vi "pointer basics.vi"() -> ()   [LabVIEW 2016]
uses:
  API/JSON Document Class/json to string/json To Minimized String - string path.vi
  API/JSON Document Class/JSON Document.lvclass
panel:
  out "error out":errorcluster
  in  "error in (no error)":errorcluster
  out "/pi":string
  out "/foo/1":string
  out "/foo/0":string
  out "/foo":string
  out "null":string
  # "Source JSON"
  # "{\n    \"foo\" : [\"bar\", \"baz\"],\n    \"pi\" : 3.1416\n}"
  # "This VI shows the basics of the pointer format.\nThe source JSON is flattened to a string at each pointer.\nrapidJSON supports String representations. Additionally, it fully supports RFC6901 also defines the URI fragment representation of JSON pointer. URI fragment is specified in RFC3986 \"Uniform Resource Identifier (URI): Generic Syntax\".\n\nThe main differences are that a the URI fragment always has a # (pound sign) in the beginning, and some characters are encoded by percent-encoding in UTF-8 sequence. For example, the following table shows different C/C++ string literals of different representations.\n\nIt additionally can accept an array of tokens"
  # "Providing the path to a key in an object return the value of that object"
  # "Providing null or an empty string returns the entire structure"
  # "Providing the path to an array element returns the element at that index"
  # "Structured types can be nested, e.g. an array inside an object."
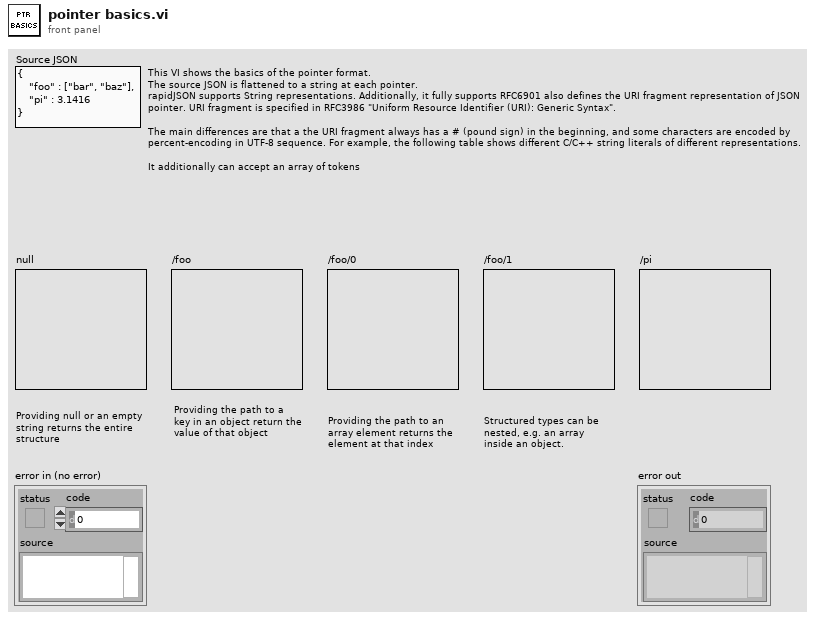
[diagram p1: front panel]
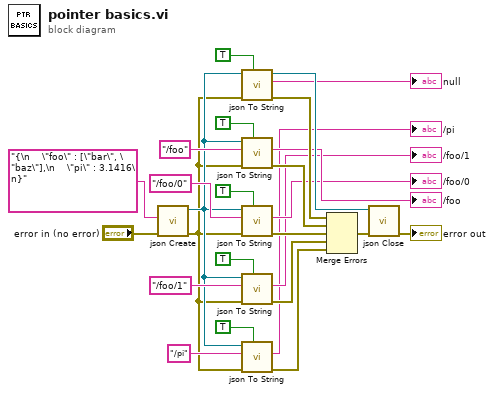
[diagram p0: block diagram]
diagram:
  n1 = call "json Create.vi"("error in (no error)"="error in (no error)", "JSON String"="{\n    \"foo\" : [\"bar\", \"baz\"],\n    \"pi\" : 3.1416\n}" ("String")) -> ("error out"=w20:errorcluster, "JSON Document out"=w21:refnum<class "JSON Document.lvclass">)  [unwired: 8 in]
  n2 = call-poly "json To String.vi"("pretty print?"=TRUE, "error in (no error)"=w20, "JSON Document in"=w21) -> ("error out"=w19:errorcluster, "json string"=→"null":string, "JSON Document out"=w13:refnum<class "JSON Document.lvclass">)  [unwired: 6 in]
  n3 = call-poly "json To String.vi"("pretty print?"=TRUE, "error in (no error)"=w20, "path"="/foo", "JSON Document in"=w21) -> ("error out"=w18:errorcluster, "json string"=→"/foo":string)  [unwired: 5 in, 1 out]
  n4 = call-poly "json To String.vi"("pretty print?"=TRUE, "error in (no error)"=w20, "path"="/foo/0", "JSON Document in"=w21) -> ("error out"=w17:errorcluster, "json string"=→"/foo/0":string)  [unwired: 5 in, 1 out]
  n5 = call-poly "json To String.vi"("pretty print?"=TRUE, "error in (no error)"=w20, "path"="/foo/1", "JSON Document in"=w21) -> ("error out"=w16:errorcluster, "json string"=→"/foo/1":string)  [unwired: 5 in, 1 out]
  n6 = call-poly "json To String.vi"("pretty print?"=TRUE, "error in (no error)"=w20, "path"="/pi", "JSON Document in"=w21) -> ("error out"=w15:errorcluster, "json string"=→"/pi":string)  [unwired: 5 in, 1 out]
  n7 = Merge Errors(w19, w18, w17, w16, w15) -> (w14:errorcluster)
  n8 = call "json Close.vi"("error in (no error)"=w14, "JSON Document in"=w13) -> ("error out"=→"error out":errorcluster)  [unwired: 9 in]
